vi "Truncate string.vi"(11 "String Path in":string) -> (3 "String path out":string)   [LabVIEW 2021]
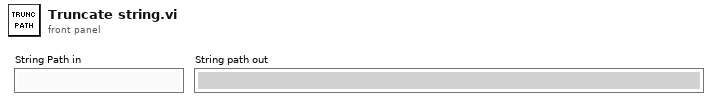
[diagram p1: front panel]
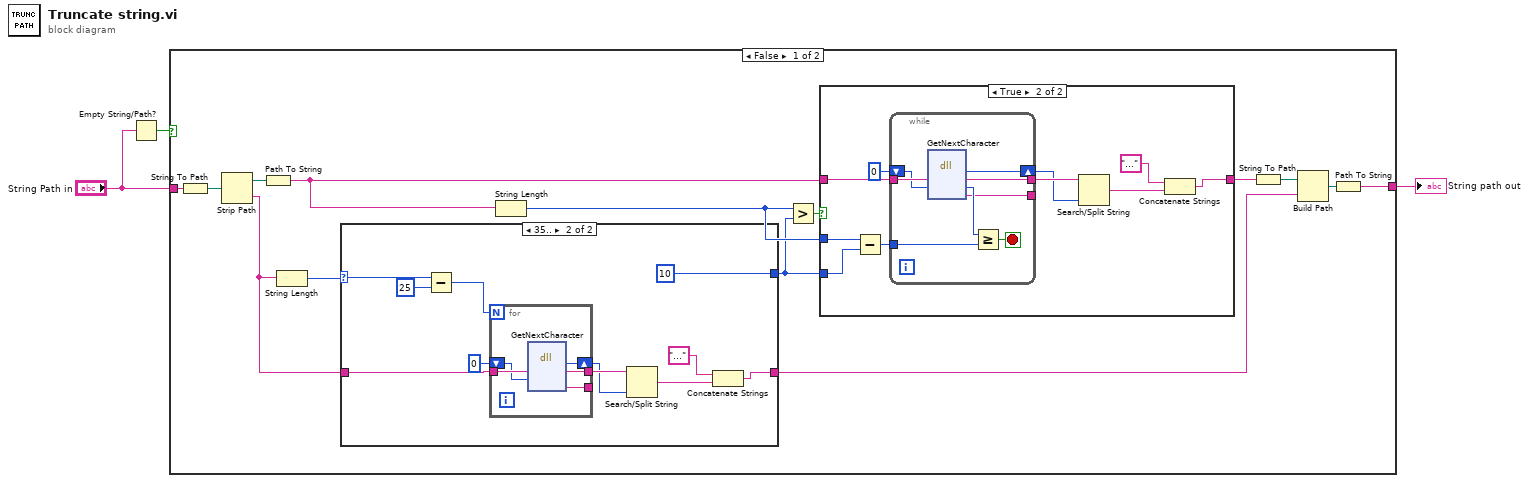
[diagram p0: block diagram]
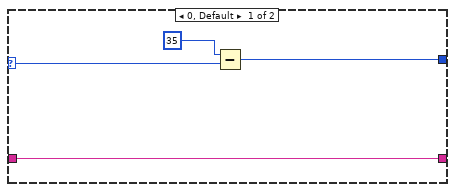
[diagram p2: hidden frame]
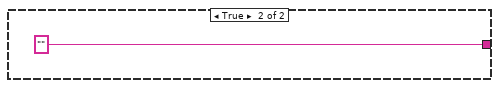
[diagram p4: hidden frame]
diagram:
  n1 = Empty String/Path?(string/path="String Path in") -> (empty?=w1:bool)
  n2 = case shown="False" w1 {
    tunnel: [w9 ""] -> w3
    tunnel: "String Path in" -> [w7 _]
    frame False {
      n3 = String To Path(string=w7) -> (path=w8:path)
      n4 = Strip Path(path=w8) -> (stripped path=w14:path, name=w5:string)
      n5 = Path To String(path=w14) -> (string=w13:string)
      n6 = String Length(string=w5) -> (length=w6:i32)
      n7 = case shown="35.." w6 {
        selector: w6 -> [w19 w24]
        tunnel: [w20 10] -> w15
        tunnel: w5 -> [w18 w30]
        tunnel: [w18 w25] -> w4
        frame 0, Default {
          n8 = Subtract(x=35 ("length"), y=w19) -> (x-y=w20:i32)
        }
        frame 35.. {
          n9 = Subtract(x=w24, y=25) -> (x-y=w22:i32)
          n10 = for {
            N: w22 -> [_]
            tunnel: [w37] -> w27
            tunnel: w30 -> [w36]
            shift-right: [w34] -> w26
            shift-left: 0 ("return type") -> [w35]
            tunnel: [w33] -> _
            n11 = dll-call lib="LabVIEW" fn="GetNextCharacter"("string"=w36, "offset"=w35) -> ("return type"=w34:i32, "string"=w37:string, "nextChar"=w33:string)  [unwired: 4 in, 3 out]
          }
          n12 = Search/Split String(string=w27, offset (0)=w26) -> (match + rest of string=w28:string)  [unwired: 3 out]
          n13 = Concatenate Strings("..." ("string"), w28) -> (w25:string)
        }
      }
      n14 = String Length(string=w13) -> (length=w16:i32)
      n15 = Greater?(x=w16, y=w15) -> (0:w17:bool)
      n16 = case shown="True" w17 {
        tunnel: w16 -> [_ w48]
        tunnel: w13 -> [w38 w43]
        tunnel: w15 -> [_ w47]
        tunnel: [w38 w45] -> w12
        frame False {
        }
        frame True {
          n17 = Subtract(x=w48, y=w47) -> (x-y=w41:i32)
          n18 = while {
            tunnel: [w56] -> w44
            tunnel: w43 -> [w55]
            shift-right: [w53] -> w40
            shift-left: 0 ("return type") -> [w54]
            tunnel: w41 -> [w51]
            tunnel: [w49] -> _
            stop <- w50 stop-if-true
            n19 = dll-call lib="LabVIEW" fn="GetNextCharacter"("string"=w55, "offset"=w54) -> ("return type"=w53:i32, "string"=w56:string, "offset"=w52:i32, "nextChar"=w49:string)  [unwired: 3 in, 3 out]
            n20 = Greater Or Equal?(x=w52, y=w51) -> (x >= y?=w50:bool)
          }
          n21 = Search/Split String(string=w44, offset (0)=w40) -> (match + rest of string=w39:string)  [unwired: 3 out]
          n22 = Concatenate Strings("..." ("string"), w39) -> (w45:string)
        }
      }
      n23 = String To Path(string=w12) -> (path=w11:path)
      n24 = Build Path(base path=w11, name or relative path=w4) -> (appended path=w10:path)
      n25 = Path To String(path=w10) -> (string=w9:string)
    }
    frame True {
    }
  }
  "String path out" <- w3
